vi "coordinatled led control panel with logging.vi"() -> ()   [LabVIEW 2013]
uses:
  Image Aquisition - Labview/Image Recorder/experiment state global.vi
panel:
  out "size of byte data":i32
  in  "stimulus value":u8
  in  "clear history":bool
  out "info":T1
  out "history":string
  in  "num bits per frame":u32=15
  in  "file name":string="900FF00.bin"
  out "byte data":u8[](array[numeric])
  in  "number of bytes":u32=450000
  in  "generate random bits":bool
  in  "update time (ms)":i32=50
  out "serial set up OK?":bool
  out "error out":errorcluster
  in  "stop":bool
  in  "Command":T2(ring)
  in  "Execute Command":bool
  in  "Teensy Serial Port Name":refnum<visa-resource-name>="COM3"
  # "60*60*1000/8 = 4.5E5 = 1 hr @ 1 kHz"
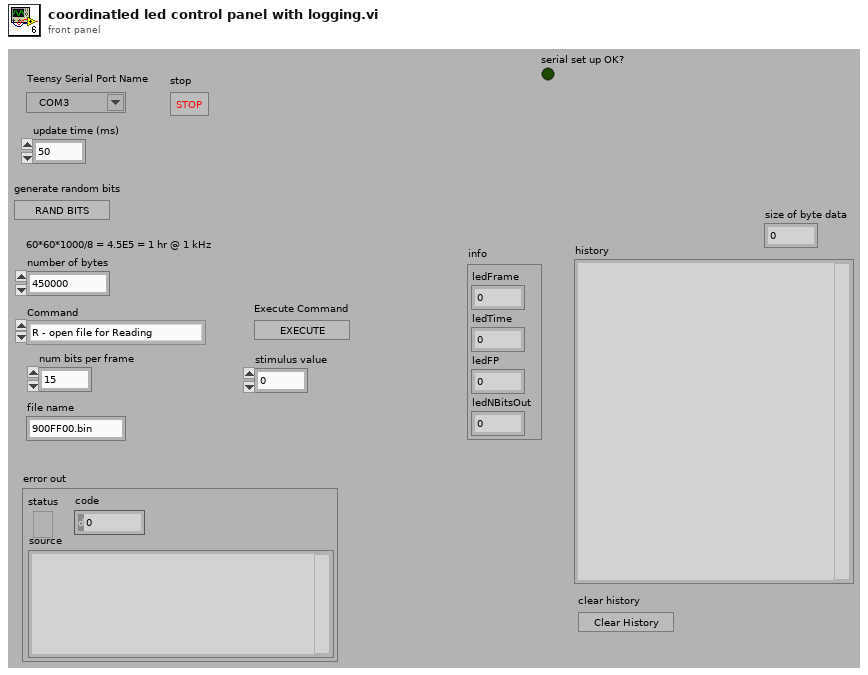
[diagram p1: front panel]
types:
  T1 = cluster{"ledFrame":i32, "ledTime":i32, "ledFP":i32, "ledNBitsOut":i32}
  T2 = enum16{"R - open file for Reading", "W - open file for Writing", "S - send bytes", "F - fetch bytes", "B - begin experiment", "E - end experiment", "N - set number of bits per frame", "I - get info", "Q - Quiet (only error msgs)", "L - Loud (acknowledge all)", "T - set stimulus state", "Y - ready to start experiment", "H - useless Help message"}
  T3 = cluster{"experiment started":bool, "experiment ended":bool, "experiment start time":u32}
  T4 = cluster{"data directory":path, "file stub":string}
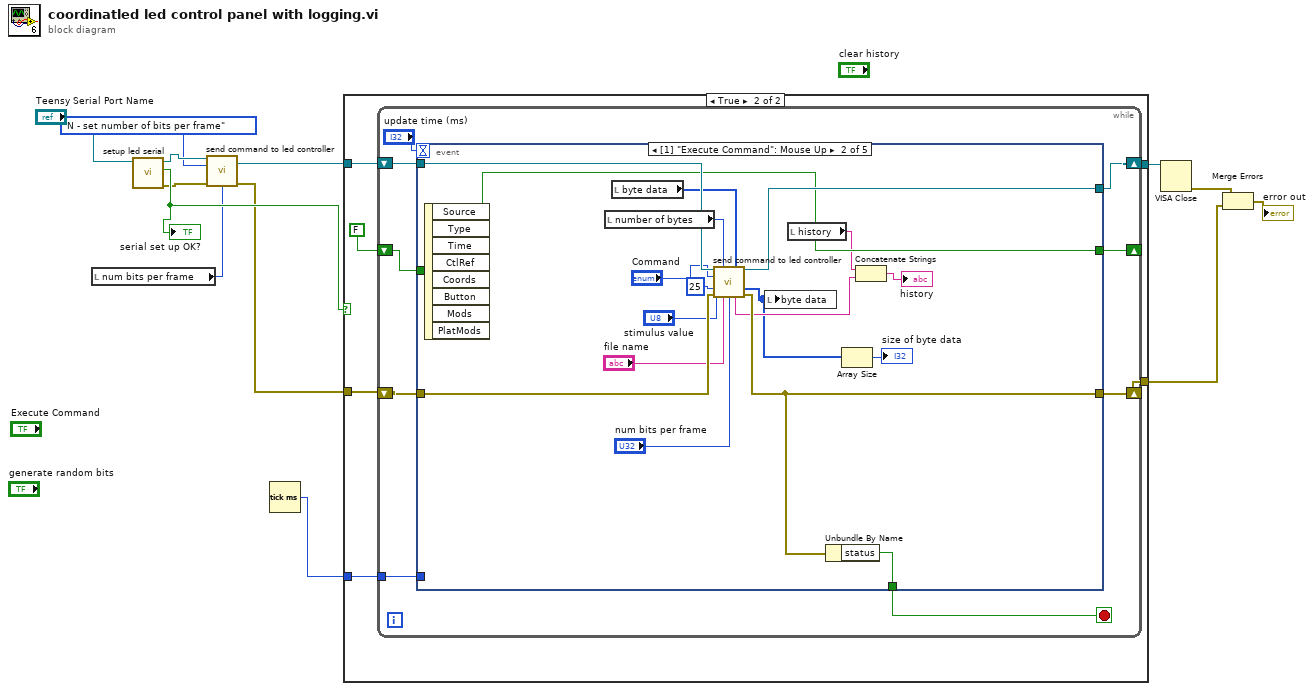
[diagram p0: block diagram]
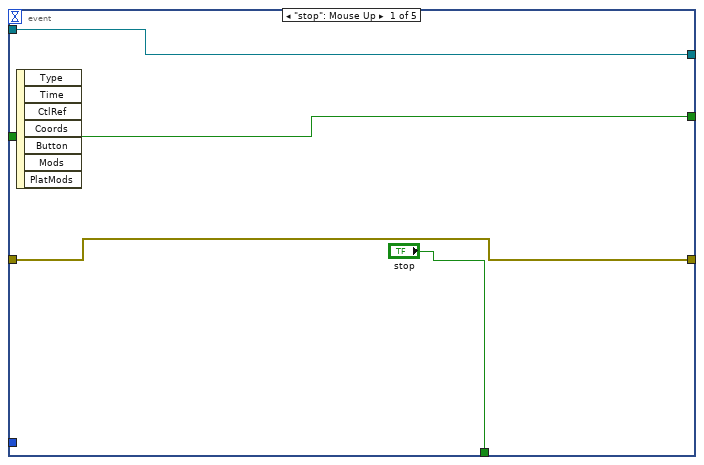
[diagram p3: hidden frame]
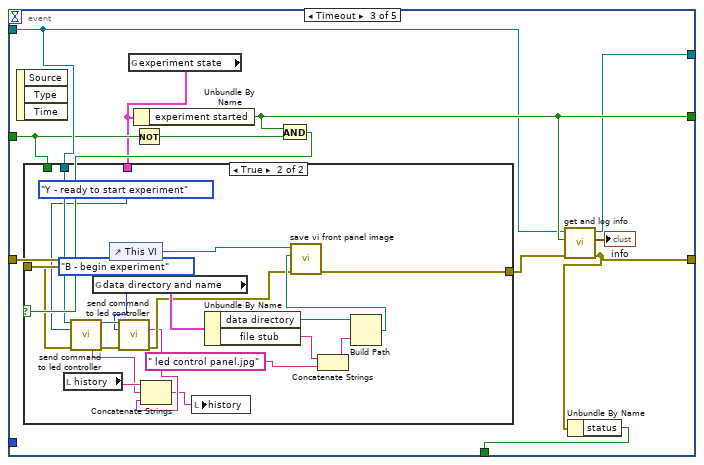
[diagram p4: hidden frame]
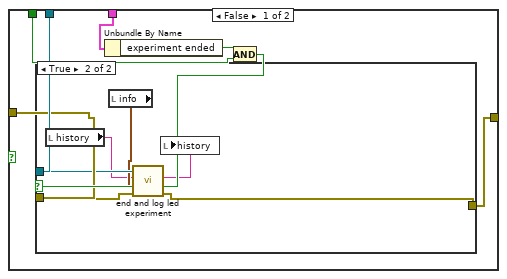
[diagram p5: hidden frame]
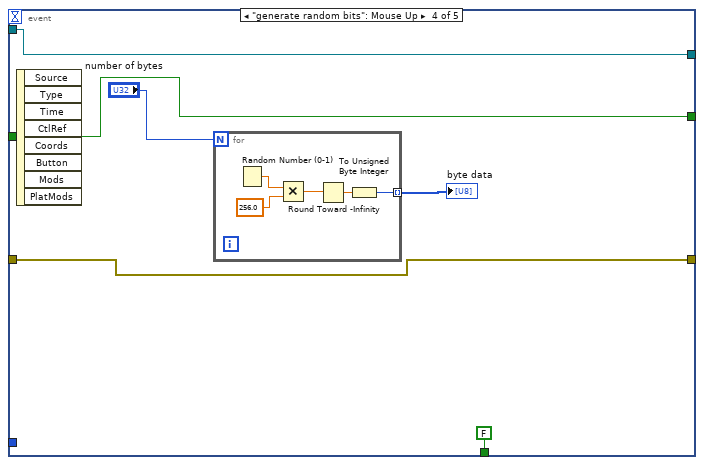
[diagram p7: hidden frame]
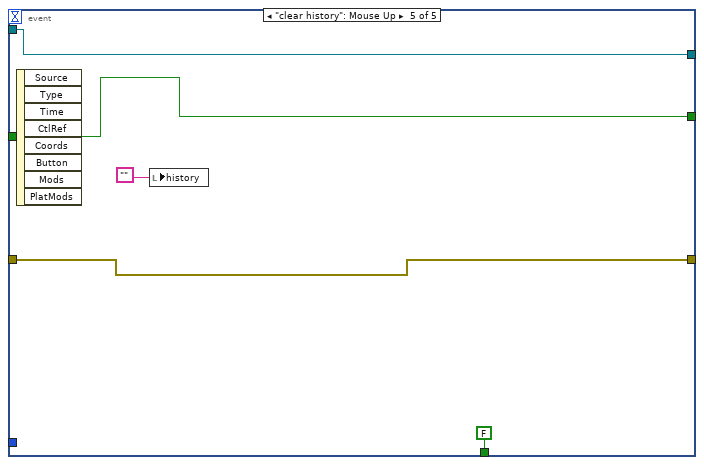
[diagram p8: hidden frame]
diagram:
  n1 = local read "num bits per frame"() -> (w1:u32)
  n2 = call "setup led serial.vi"("Teensy Serial Port"="Teensy Serial Port Name") -> ("error out"=w6:errorcluster, "OK"=w8:bool, "Teensy Serial Port"=w4:refnum<visa-resource-name>)  [unwired: 8 in]
  "serial set up OK?" <- w8
  n3 = call "send command to led controller.vi"("Teensy Serial Port"=w4, "Command"=T2."N - set number of bits per frame", "error in"=w6, "num bits per frame"=w1) -> ("teensy serial port out"=w3:refnum<visa-resource-name>, "error out"=w5:errorcluster)  [unwired: 6 in, 4 out]
  n4 = Tick Count (ms)() -> (millisecond timer value=w7:u32)
  n5 = case shown="True" w8 {
    tunnel: [w15 w21] -> w12
    tunnel: [w14 w20] -> w10
    tunnel: w5 -> [w14 w19]
    tunnel: w3 -> [w15 w18]
    tunnel: w7 -> [_ w16]
    frame False {
    }
    frame True {
      n6 = while {
        shift-right: [w29] -> w20
        shift-left: w19 -> [w30]
        shift-right: [w26] -> w21
        shift-left: w18 -> [w28]
        shift-right: [w24] -> _
        shift-left: FALSE ("experiment started") -> [w23]
        tunnel: w16 -> [w22]
        stop <- w27 stop-if-true
        n7 = event shown="[1] \"Execute Command\": Mouse Up" {
          selector: _ -> [_ _ _ _ _]
          dyn-events: _ -> [_ _ _ _ _]
          timeout: "update time (ms)" -> [_ _ _ _ _]
          tunnel: w30 -> [w33 w52 w63 w101 w112]
          tunnel: [w33 w47 w59 w101 w112] -> w29
          tunnel: w28 -> [w32 w51 w55 w100 w111]
          tunnel: [w32 w50 w57 w100 w111] -> w26
          tunnel: ["stop" w46 w61 FALSE ("status") FALSE ("status")] -> w27
          tunnel: [w31 w48 w58 w99 w110] -> w24
          tunnel: w23 -> [w31 w48 w54 w99 w110]
          tunnel: w22 -> [_ _ _ _ _]
          event "stop": Mouse Up {
            n8 = event-data() -> ()  [unwired: 1 in, 7 out]
          }
          event "Execute Command": Mouse Up {
            n9 = event-data() -> ()  [unwired: 1 in, 8 out]
            n10 = local read "number of bytes"() -> (w44:u32)
            n11 = local read "byte data"() -> (w43:u8[])
            n12 = call "send command to led controller.vi"("Teensy Serial Port"=w51, "num bytes to read"=w44, "bytes to send"=w43, "Command"="Command", "stimulus value"="stimulus value", "milliseconds to wait between write and read"=u32 25, "error in"=w52, "file name"="file name", "num bits per frame"="num bits per frame") -> ("teensy serial port out"=w50:refnum<visa-resource-name>, "bytes read"=w36:u8[], "command and response with time"=w39:string, "error out"=w47:errorcluster)  [unwired: 1 in, 2 out]
            n13 = local write "byte data"(w36) -> ()
            n14 = local read "history"() -> (w40:string)
            n15 = Unbundle By Name(w47) -> ("status"=w46:bool)
            n16 = Array Size(array=w36) -> (size(s)=→"size of byte data":i32)
            n17 = Concatenate Strings(w40, w39) -> (→"history":string)
          }
          event Timeout {
            n18 = event-data() -> ()  [unwired: 1 in, 3 out]
            n19 = global read "experiment state global.vi" "experiment state"() -> (w53:T3)
            n20 = Unbundle By Name(w53) -> ("experiment started"=w58:bool)
            n21 = Not(x=w54) -> (.not. x?=w64:bool)
            n22 = And(x=w58, y=w64) -> (x .and. y?=w62:bool)
            n23 = case shown="True" w62 {
              tunnel: w63 -> [w66 w89]
              tunnel: [w65 w81] -> w60
              tunnel: w55 -> [w67 w92]
              tunnel: w54 -> [w69 _]
              tunnel: w53 -> [w71 _]
              frame False {
                n24 = Unbundle By Name(w71) -> ("experiment ended"=w70:bool)
                n25 = And(x=w70, y=w69) -> (x .and. y?=w68:bool)
                n26 = case shown="True" w68 {
                  tunnel: w67 -> [_ w76]
                  tunnel: w66 -> [w72 w78]
                  tunnel: [w72 w77] -> w65
                  frame False {
                  }
                  frame True {
                    n27 = local read "history"() -> (w74:string)
                    n28 = local read "info"() -> (w75:T1)
                    n29 = call "end and log led experiment.vi"("error in"=w78, "info"=w75, "history"=w74, "Teensy Serial Port"=w76) -> ("error out"=w77:errorcluster, "history out"=w73:string)  [unwired: 5 in, 1 out]
                    n30 = local write "history"(w73) -> ()
                  }
                }
              }
              frame True {
                n31 = local read "history"() -> (w86:string)
                n32 = call "send command to led controller.vi"("Teensy Serial Port"=w92, "Command"=T2."Y - ready to start experiment", "error in"=w89) -> ("teensy serial port out"=w91:refnum<visa-resource-name>, "command and response with time"=w85:string, "error out"=w93:errorcluster)  [unwired: 7 in, 3 out]
                n33 = global read "experiment state global.vi" "data directory and name"() -> (w96:T4)
                n34 = control-ref of="This VI"() -> (w97:refnum<vi>)
                n35 = call "send command to led controller.vi"("Teensy Serial Port"=w91, "Command"=T2."B - begin experiment", "error in"=w93) -> ("response"=w84:string, "error out"=w88:errorcluster)  [unwired: 7 in, 4 out]
                n36 = Concatenate Strings(w86, w85, w84) -> (w83:string)
                n37 = local write "history"(w83) -> ()
                n38 = Unbundle By Name(w96) -> ("data directory"=w82:path, "file stub"=w80:string)
                n39 = Concatenate Strings(w80, " led control panel.jpg" ("string")) -> (w95:string)
                n40 = Build Path(base path=w82, name or relative path=w95) -> (appended path=w94:path)
                n41 = call "save vi front panel image.vi"("error in (no error)"=w88, "path to JPEG file"=w94, "This VI"=w97) -> ("error out"=w81:errorcluster)  [unwired: 8 in]
              }
            }
            n42 = call "get and log info.vi"("error in"=w60, "log data?"=w58, "Teensy Serial Port"=w55) -> ("error out"=w59:errorcluster, "info"=→"info":T1, "LADY GAGA v2 Serial Port out"=w57:refnum<visa-resource-name>)  [unwired: 6 in]
            n43 = Unbundle By Name(w59) -> ("status"=w61:bool)
          }
          event "generate random bits": Mouse Up {
            n44 = event-data() -> ()  [unwired: 1 in, 8 out]
            n45 = for {
              N: "number of bytes" -> [_]
              tunnel: [w104] -> w103 mode=indexing
              n46 = Random Number (0-1)() -> (number: 0 to 1=w108:dbl)
              n47 = Multiply(x=w108, y=256.0) -> (x*y=w106:dbl)
              n48 = Round Toward -Infinity(1:w106) -> (0:w105:dbl)
              n49 = To Unsigned Byte Integer(number=w105) -> (unsigned 8bit integer=w104:u8)
            }
            "byte data" <- w103
          }
          event "clear history": Mouse Up {
            n50 = event-data() -> ()  [unwired: 1 in, 8 out]
            n51 = local write "history"("") -> ()
          }
        }
      }
    }
  }
  n52 = VISA Close(VISA resource name=w12) -> (error out=w11:errorcluster)  [unwired: 1 in]
  n53 = Merge Errors(w11, w10) -> (→"error out":errorcluster)
